vi "StrToHex.vi"(1 "StrIn":string) -> (0 "StrOut":string)   [LabVIEW 2013]
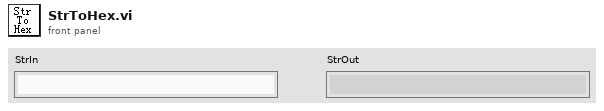
[diagram p1: front panel]
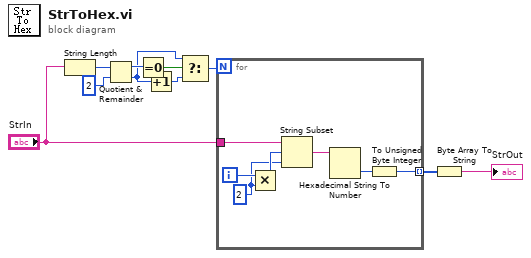
[diagram p0: block diagram]
diagram:
  n1 = String Length(string="StrIn") -> (length=w10:i32)
  n2 = Quotient & Remainder(x=w10, y=2) -> (x-y*floor(x/y)=w8:i32, floor(x/y)=w6:i32)
  n3 = Equal To 0?(x=w8) -> (x = 0?=w7:bool)
  n4 = Increment(x=w6) -> (x+1=w5:i32)
  n5 = Select(t=w6, s=w7, f=w5) -> (s? t:f=w4:i32)
  n6 = for {
    N: w4 -> [_]
    tunnel: "StrIn" -> [w17]
    tunnel: [w11] -> w2 mode=indexing
    i -> [w16]
    w14 = 2
    n7 = Multiply(x=w16, y=w14) -> (x*y=w15:i32)
    n8 = String Subset(string=w17, offset (0)=w15, length (rest)=w14) -> (substring=w13:string)
    n9 = Hexadecimal String To Number(string=w13) -> (number=w12:u32)  [unwired: 2 in, 1 out]
    n10 = To Unsigned Byte Integer(number=w12) -> (unsigned 8bit integer=w11:u8)
  }
  n11 = Byte Array To String(unsigned byte array=w2) -> (string=→"StrOut":string)
